vi "Read Interval from SnP File.vi"(0 "Result File Path In":path, 11 "error in":errorcluster) -> (4 "Result File Path Out":path, 6 "Interval":i32, 15 "error out":errorcluster)   [LabVIEW 2023, in "RFFixtureCharact.RFPM.lvlib" / "Charact Result Accessor.lvclass"]
uses:
  Charact Result Accessor.lvclass
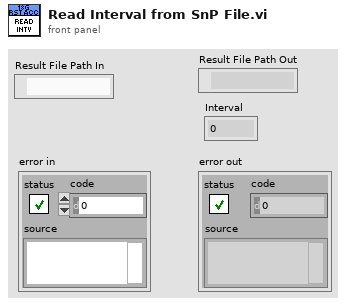
[diagram p1: front panel]
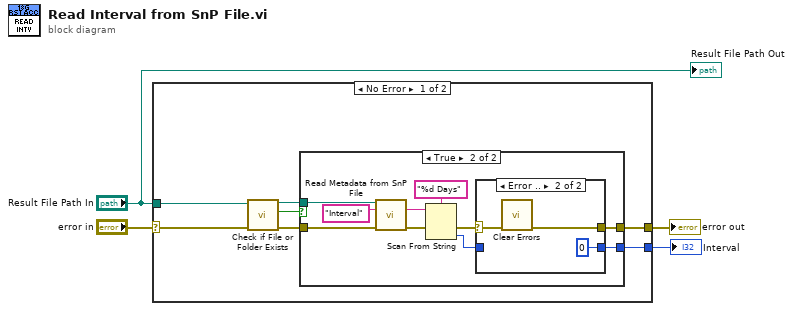
[diagram p0: block diagram]
diagram:
  n1 = case shown="No Error" "error in" {
    selector: "error in" -> [w6 w28]
    tunnel: [w11 w28] -> w3
    tunnel: [w7 _] -> w2
    tunnel: "Result File Path In" -> [w5 _]
    frame No Error {
      n2 = call <vilib>:"Check if File or Folder Exists.vi"("error in (no error)"=w6, "path"=w5) -> ("error out"=w9:errorcluster, "file or folder exists?"=w8:bool, "dup path"=w10:path)  [unwired: 7 in]
      n3 = case shown="True" w8 {
        tunnel: [w12 w15] -> w11
        tunnel: w10 -> [_ w18]
        tunnel: w9 -> [w12 w17]
        tunnel: [_ w14] -> w7
        frame False {
        }
        frame True {
          n4 = call "Read Metadata from SnP File.vi"("SnP File Path in"=w18, "Key"="Interval", "error in (no error)"=w17) -> ("Value"=w20:string, "error out"=w21:errorcluster)  [unwired: 10 in, 1 out]
          n5 = Scan From String(format string="%d Days", input string=w20, error in=w21) -> (error out=w16:errorcluster, output 1=w13:i32)  [unwired: 2 in, 2 out]
          n6 = case shown="Error .." w16 {
            selector: w16 -> [w24 w27]
            tunnel: [w24 w26] -> w15
            tunnel: [w23 0] -> w14
            tunnel: w13 -> [w23 _]
            frame No Error {
            }
            frame Error {
              n7 = call <vilib>:"Clear Errors.vi"("error in (no error)"=w27) -> ("error out"=w26:errorcluster)  [unwired: 5 in, 1 out]
            }
          }
        }
      }
    }
    frame Error {
    }
  }
  "error out" <- w3
  "Interval" <- w2
  "Result File Path Out" <- "Result File Path In"
